vi "PH_AxisGUI_BaseClass.PC_Settings.vi"(0 "i ref in":refnum<vi>, 2 "Service Name":string="N/A", 3 "Axis Settings":T1={"Sign change"=FALSE, "Width"=0.0, "Calibration"=0.0, "Unit"="Steps", "Motor Type"=enum."Unspecific", "Unit Width"="", "Unit CF"=""}, 4 "No Link?":bool, 5 "error in":errorcluster) -> (14 "i ref out":refnum<vi>, 16 "Axis":i32=-1, 19 "error":errorcluster)   [LabVIEW 2014, in "PH_AxisGUI_BaseClass.lvlib"]
doc: "This VI deals with information given by an axis."
uses:
  PH_AxisGUI_BaseClass.lvlib
  PH_Stepmotor_BaseClass/PH_Stepmotor_BaseClass.Axis Settings.ctl
  PH_Stepmotor_BaseClass/PH_Stepmotor_BaseClass.Motor Type.ctl
  PH_Stepmotor_BaseClass/PH_Stepmotor_BaseClass.Axis DIM Tags.ctl
  PH_Stepmotor_BaseClass/PH_Stepmotor_BaseClass.lvlib
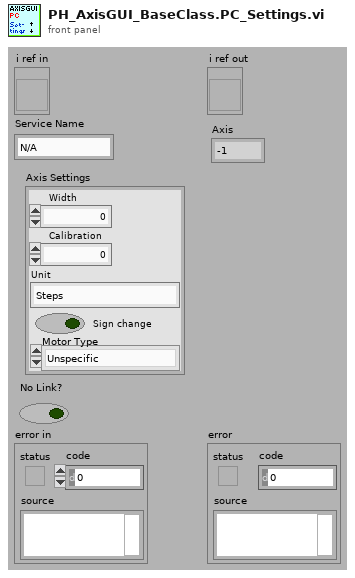
[diagram p1: front panel]
types:
  T1 = typedef "PH_Stepmotor_BaseClass.lvlib/PH_Stepmotor_BaseClass.Axis Settings.ctl" = cluster{"Sign change":bool, "Width":dbl, "Calibration":dbl, "Unit":string, "Motor Type":T2, "Unit Width":string, "Unit CF":string}
  T2 = typedef "PH_Stepmotor_BaseClass.lvlib/PH_Stepmotor_BaseClass.Motor Type.ctl" = enum16{"Unspecific", "OWIS 49.120.2633", "OWIS 49.060.1033", "OWIS 43.040.2558", "Diamond Motion 2200 series", "OWIS 49.120.266B.MV6", "Calorimeter", "Linear Stage 1", "MICOS VT-80", "MICOS VT-80 S", "Standa Rotstage nt0.95A", "PUF RA 320.200", "PUF RA 800.200", "PUF RA 800.400", "PUF RA 400.50", "1324.nn.800.50", "1324.n9c.800.50", "1324.nn.320.200", "1324.nn.400.200", "1324.nn.800.200", "1324.nn.400.50", "1324.8c9c.800.50", "1324.8c9c.400.200"}
  T3 = typedef "PH_Stepmotor_BaseClass.lvlib/PH_Stepmotor_BaseClass.Axis DIM Tags.ctl" = enum16{"no Info", "Information", "Settings"}
  T4 = typedef "PH_AxisGUI_BaseClass.lvlib/PH_AxisGUI_BaseClass.Axis Attributes.ctl" = cluster{"Axis GUI Refs":T5, "Address":T6, "Name":string, "Label \"Back\"":string, "Labell \"Forth\"":string, "Moving?":bool}
  T5 = typedef "PH_AxisGUI_BaseClass.lvlib/PH_AxisGUI_BaseClass.Axis GUI Refs.ctl" = cluster{"Back":refnum<vi>, "Forth":refnum<vi>, "Status":refnum<vi>, "Target":refnum<vi>, "Address":refnum<vi>, "Status Bar":refnum<vi>, "Settings":refnum<vi>, "Activity":refnum<vi>, "Clear Error":refnum<vi>}
  T6 = typedef "PH_Stepmotor_BaseClass.lvlib/PH_Stepmotor_BaseClass.Axis Address.ctl" = cluster{"Instance":string, "Motor Nr":i32}
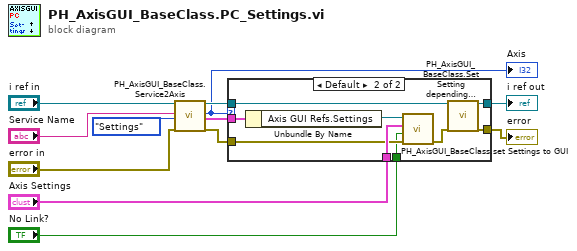
[diagram p0: block diagram]
diagram:
  n1 = call "PH_AxisGUI_BaseClass.Service2Axis.vi"("i ref in"="i ref in", "Service Name"="Service Name", "Tag"=PH_Stepmotor_BaseClass.Axis_DIM_Tags."Settings", "error in"="error in") -> ("i ref out"=w6:refnum<vi>, "Axis"=w2:i32, "Axis Data"=w4:T4, "error out"=w5:errorcluster)  [unwired: 12 in]
  "Axis" <- w2
  n2 = case shown="Default" w2 {
    tunnel: [w13 w23] -> w12
    tunnel: [w14 w22] -> w10
    tunnel: "Axis Settings" -> [_ w20]
    tunnel: w6 -> [w14 w19]
    tunnel: w5 -> [w13 w18]
    tunnel: w4 -> [_ w17]
    tunnel: "No Link?" -> [_ w15]
    frame -1 {
    }
    frame Default {
      n3 = Unbundle By Name(w17) -> ("Axis GUI Refs.Settings"=w16:refnum<vi>)
      n4 = call "PH_AxisGUI_BaseClass.set Settings to GUI.vi"("error in (no error)"=w18, "No link?"=w15, "Axis Settings"=w20, "GUI Ref Settings"=w16) -> ("error out"=w21:errorcluster)  [unwired: 3 in]
      n5 = call "PH_AxisGUI_BaseClass.Set Setting depending Captions.vi"("i ref out"=w19, "error in"=w21) -> ("i ref out"=w22:refnum<vi>, "error out"=w23:errorcluster)  [unwired: 16 in]
    }
  }
  "error" <- w12
  "i ref out" <- w10
